vi "HCl_volume_global.vi"() -> ()   [LabVIEW 2010]
panel:
  out "HCl Volume (uncorr)":dbl
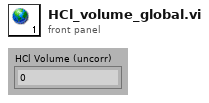
[diagram p1: front panel]
diagram:
